vi "test_number_selector.vi"(0 "1st tst in":dbl, 2 "2nd tst in":dbl, 3 "tst mod":string) -> (5 "1st tst out":dbl, 6 "2nd tst out":dbl)   [LabVIEW 2015]
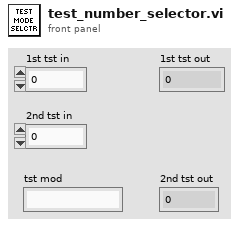
[diagram p1: front panel]
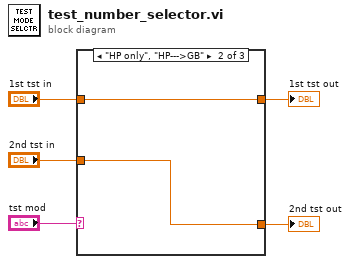
[diagram p0: block diagram]
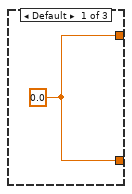
[diagram p2: hidden frame]
diagram:
  n1 = case shown="\"HP only\", \"HP--->GB\"" "tst mod" {
    tunnel: "1st tst in" -> [_ w8 w10]
    tunnel: "2nd tst in" -> [_ w7 w9]
    tunnel: [w6 w8 w9] -> w2
    tunnel: [w6 w7 w10] -> w1
    frame Default {
      w6 = 0.0
    }
    frame "HP only", "HP--->GB" {
    }
    frame "GB only", "GB--->HP" {
    }
  }
  "1st tst out" <- w2
  "2nd tst out" <- w1
